vi "S2C_FORNAX_Poly_EmA2dCalDataCommand.vi"(8 "Error In":errorcluster, 10 "EmA2dCalDataCommand":T3={"Partition"="Default", "Message"="EmA2dCalDataCommand", "M_Command"=0, "M_CalibrationType"=0, "M_CalibrationTime"="", "M_Options"="", "M_EmA2dCalData.M_MonoLowVoltPrimary.M_Offset"=0.0, "M_EmA2dCalData.M_MonoLowVoltPrimary.M_Gain"=0.0, "M_EmA2dCalData.M_MonoLowVoltSecondary.M_Offset"=0.0, "M_EmA2dCalData.M_MonoLowVoltSecondary.M_Gain"=0.0, "M_EmA2dCalData.M_MonoHighVoltPrimary.M_Offset"=0.0, "M_EmA2dCalData.M_MonoHighVoltPrimary.M_Gain"=0.0, "M_EmA2dCalData.M_MonoHighVoltSecondary.M_Offset"=0.0, "M_EmA2dCalData.M_MonoHighVoltSecondary.M_Gain"=0.0, "M_EmA2dCalData.M_BipLowVoltPrimary.M_Offset"=0.0, "M_EmA2dCalData.M_BipLowVoltPrimary.M_Gain"=0.0, "M_EmA2dCalData.M_BipLowVoltSecondary.M_Offset"=0.0, "M_EmA2dCalData.M_BipLowVoltSecondary.M_Gain"=0.0, "M_EmA2dCalData.M_BipHighVoltPrimary.M_Offset"=0.0, "M_EmA2dCalData.M_BipHighVoltPrimary.M_Gain"=0.0, "M_EmA2dCalData.M_BipHighVoltSecondary.M_Offset"=0.0, "M_EmA2dCalData.M_BipHighVoltSecondary.M_Gain"=0.0, "M_EmA2dCalData.M_BipLowCurrentPrimary.M_Offset"=0.0, "M_EmA2dCalData.M_BipLowCurrentPrimary.M_Gain"=0.0, "M_EmA2dCalData.M_BipLowCurrentSecondary.M_Offset"=0.0, "M_EmA2dCalData.M_BipLowCurrentSecondary.M_Gain"=0.0, "M_EmA2dCalData.M_BipHighCurrentPrimary.M_Offset"=0.0, "M_EmA2dCalData.M_BipHighCurrentPrimary.M_Gain"=0.0, "M_EmA2dCalData.M_BipHighCurrentSecondary.M_Offset"=0.0, "M_EmA2dCalData.M_BipHighCurrentSecondary.M_Gain"=0.0} {"M_CalibrationType" items=["CALIBRATION_TYPE_FIELD"=0, "CALIBRATION_TYPE_FACTORY"=1, "CALIBRATION_TYPE_UNKNOWN"=-1]; "M_Command" items=["LOG_COMMAND_INVALID", "LOG_COMMAND_CLEAR_ALL", "LOG_COMMAND_CLEAR_EVENT", "LOG_COMMAND_CLEAR_ALARM", "LOG_COMMAND_CLEAR_RFID", "LOG_COMMAND_ROTATE_ALL", "LOG_COMMAND_ROTATE_EVENT", "LOG_COMMAND_ROTATE_ALARM", "LOG_COMMAND_ROTATE_RFID", "LOG_COMMAND_CLEAR_RFDATA", "LOG_COMMAND_RF_DATA_ALL_MODES", "LOG_COMMAND_RF_DATA_LIGASURE_ONLY", "LOG_COMMAND_CLEAR_USAGE", "LOG_COMMAND_ROTATE_USAGE", "NUM_LOG_COMMANDS"]}, 11 "Settings":T4={"Driver"="Fornax", "Command"="EmA2dCalDataCommand", "Return"="ErrorStatus", "Parameters"="", "Timeout"=10.0}) -> (0 "Error Out":errorcluster, 3 "Response":string)   [LabVIEW 2015]
uses:
  Typedefs/LogCommand.ctl
  Typedefs/CalibrationType.ctl
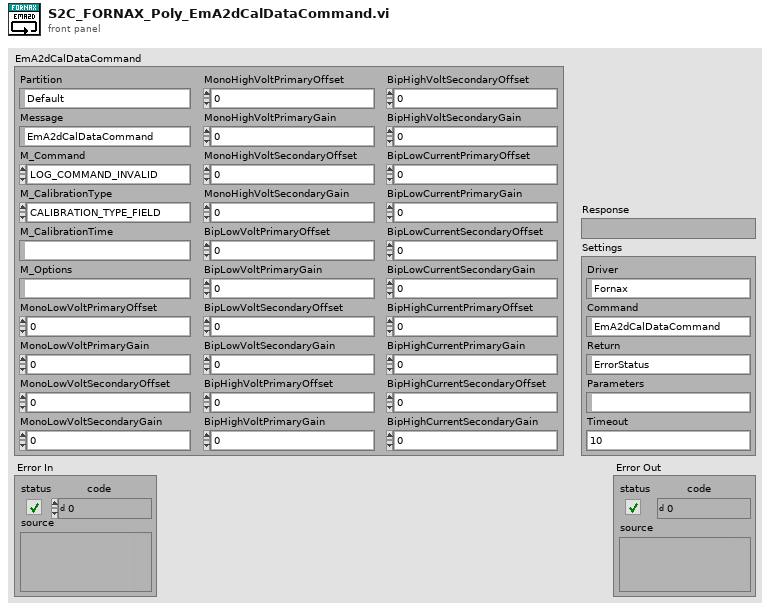
[diagram p1: front panel]
types:
  T1 = typedef "LogCommand.ctl" = i16
  T2 = typedef "CalibrationType.ctl" = i16
  T3 = cluster{"Partition":string, "Message":string, "M_Command":T1, "M_CalibrationType":T2, "M_CalibrationTime":string, "M_Options":string, "M_EmA2dCalData.M_MonoLowVoltPrimary.M_Offset":dbl, "M_EmA2dCalData.M_MonoLowVoltPrimary.M_Gain":dbl, "M_EmA2dCalData.M_MonoLowVoltSecondary.M_Offset":dbl, "M_EmA2dCalData.M_MonoLowVoltSecondary.M_Gain":dbl, "M_EmA2dCalData.M_MonoHighVoltPrimary.M_Offset":dbl, "M_EmA2dCalData.M_MonoHighVoltPrimary.M_Gain":dbl, "M_EmA2dCalData.M_MonoHighVoltSecondary.M_Offset":dbl, "M_EmA2dCalData.M_MonoHighVoltSecondary.M_Gain":dbl, "M_EmA2dCalData.M_BipLowVoltPrimary.M_Offset":dbl, "M_EmA2dCalData.M_BipLowVoltPrimary.M_Gain":dbl, "M_EmA2dCalData.M_BipLowVoltSecondary.M_Offset":dbl, "M_EmA2dCalData.M_BipLowVoltSecondary.M_Gain":dbl, "M_EmA2dCalData.M_BipHighVoltPrimary.M_Offset":dbl, "M_EmA2dCalData.M_BipHighVoltPrimary.M_Gain":dbl, "M_EmA2dCalData.M_BipHighVoltSecondary.M_Offset":dbl, "M_EmA2dCalData.M_BipHighVoltSecondary.M_Gain":dbl, "M_EmA2dCalData.M_BipLowCurrentPrimary.M_Offset":dbl, "M_EmA2dCalData.M_BipLowCurrentPrimary.M_Gain":dbl, "M_EmA2dCalData.M_BipLowCurrentSecondary.M_Offset":dbl, "M_EmA2dCalData.M_BipLowCurrentSecondary.M_Gain":dbl, "M_EmA2dCalData.M_BipHighCurrentPrimary.M_Offset":dbl, "M_EmA2dCalData.M_BipHighCurrentPrimary.M_Gain":dbl, "M_EmA2dCalData.M_BipHighCurrentSecondary.M_Offset":dbl, "M_EmA2dCalData.M_BipHighCurrentSecondary.M_Gain":dbl}
  T4 = cluster{"Driver":string, "Command":string, "Return":string, "Parameters":string, "Timeout":dbl}
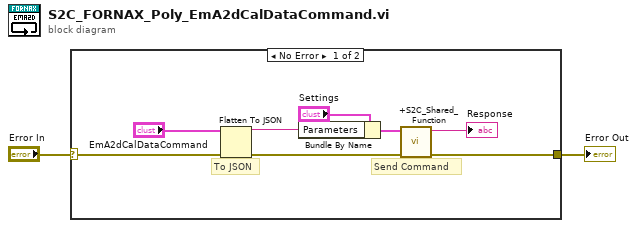
[diagram p0: block diagram]
diagram:
  n1 = case shown="No Error" "Error In" {
    selector: "Error In" -> [w6 w11]
    tunnel: [w5 w11] -> w1
    frame No Error {
      # "To JSON"
      # "Send Command"
      n2 = Flatten To JSON(anything="EmA2dCalDataCommand", error in (no error)=w6) -> (JSON string=w7:string, 11:w9:errorcluster)  [unwired: 1 in]
      n3 = Bundle By Name(cluster="Settings", "Parameters"=w7) -> (w10:T4)
      n4 = call "+S2C_Shared_Function.vi"("Error In"=w9, "Settings"=w10) -> ("Error Out"=w5:errorcluster, "Response"=→"Response":string)  [unwired: 8 in]
    }
    frame Error {
    }
  }
  "Error Out" <- w1
